vi "报警信息.vi"() -> ()   [LabVIEW 2020]
panel:
  out "报警信息":string[][](table)
  # "报警信息"
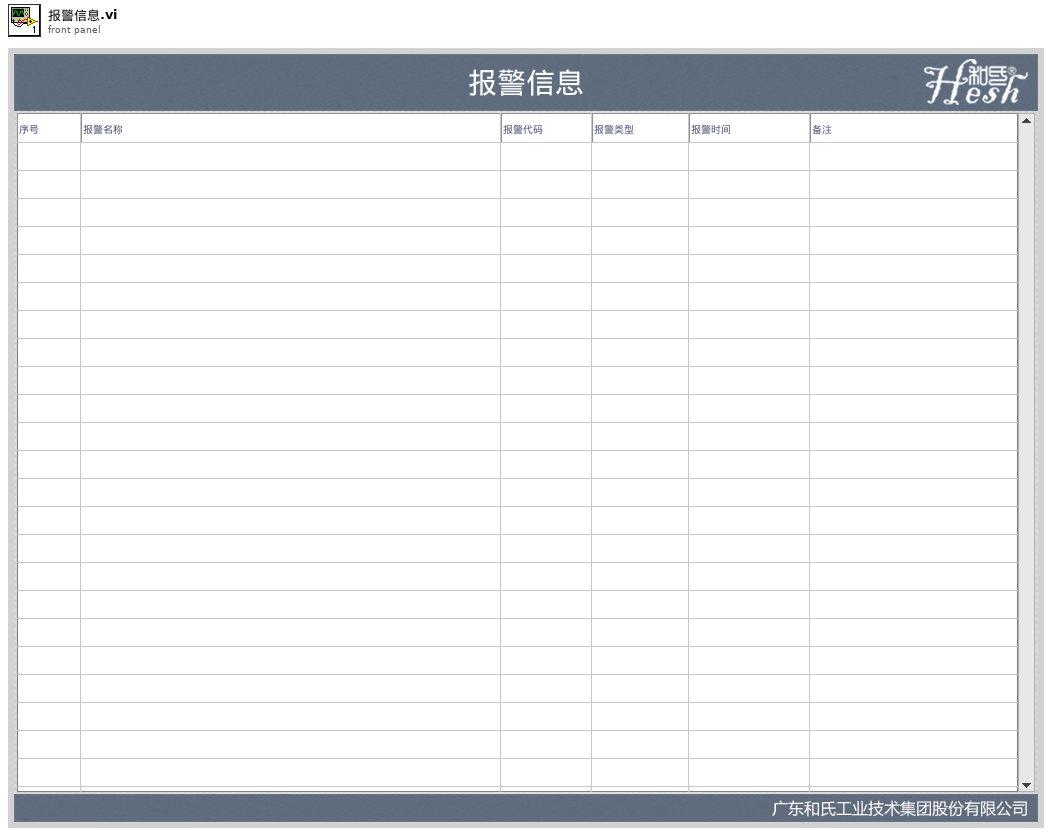
[diagram p1: front panel]
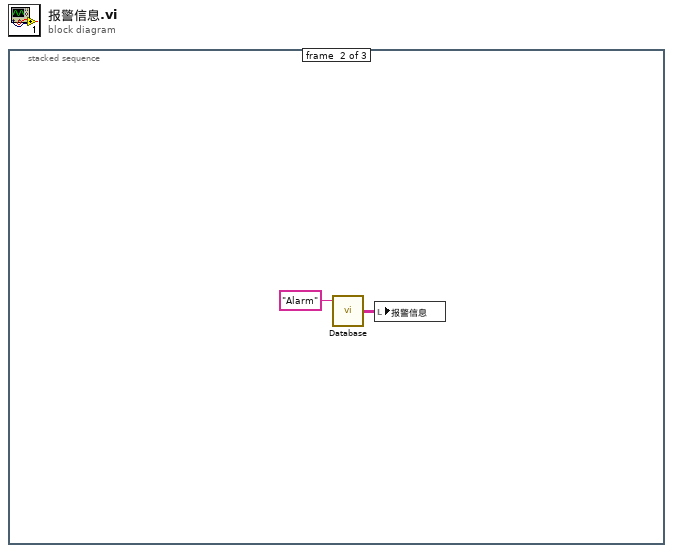
[diagram p0: block diagram]
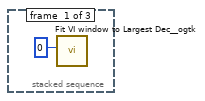
[diagram p2: hidden frame]
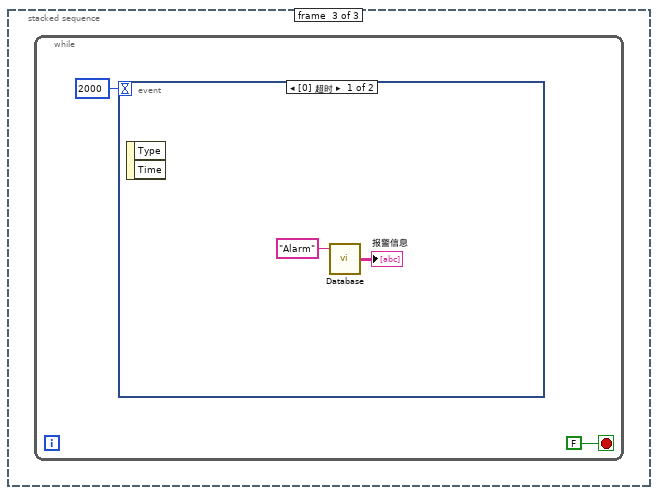
[diagram p3: hidden frame]
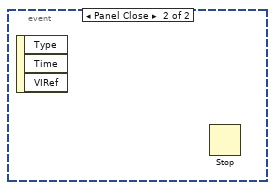
[diagram p4: hidden frame]
diagram:
  n1 = stacked-sequence {
    frame #0 {
      n2 = call <userlib>:"Fit VI window to Largest Dec__ogtk.vi"("border spacing (2 px)"=0) -> ()  [unwired: 5 in, 2 out]
    }
    frame #1 {
      n3 = call "Database.vi"("table"="Alarm") -> ("data"=w3:string[][])  [unwired: 2 in, 2 out]
      n4 = local write "报警信息"(w3) -> ()
    }
    frame #2 {
      n5 = while {
        stop <- FALSE stop-if-true
        n6 = event shown="[0] 超时" {
          selector: _ -> [_ _]
          dyn-events: _ -> [_ _]
          timeout: 2000 -> [_ _]
          event Timeout {
            n7 = event-data() -> ()  [unwired: 1 in, 2 out]
            n8 = call "Database.vi"("table"="Alarm") -> ("data"=→"报警信息":string[][])  [unwired: 2 in, 2 out]
          }
          event Panel Close {
            n9 = event-data() -> ()  [unwired: 1 in, 3 out]
            n10 = Stop() -> ()  [unwired: 1 in]
          }
        }
      }
    }
  }
